vi "Redefine Master.vi"(8 "error in (no error)":errorcluster, 11 "MB_TCP in":refnum<class "Modbus Master CR.lvclass">) -> (0 "error out":errorcluster, 3 "MB_TCP out":refnum<class "Modbus Master CR.lvclass">)   [LabVIEW 2021, in "Modbus Master CR.lvclass"]
uses:
  Modbus Master CR.lvclass
  D:/my_projects/projects/Algorithms/Labview/21/Modbus_v121c/Network Protocol/Network Protocol.lvclass
  Network Protocol.lvclass/Network Protocol.ctl
  Modbus Master CR.lvclass/Modbus Master CR.ctl
  MB Param/MBTCP Param/MBTCP Param.lvclass
  Transmission Data Unit/IP/IP Data Unit.lvclass
  D:/my_projects/projects/Algorithms/Labview/21/Modbus_v121c/Transmission Data Unit/Transmission Data Unit.lvclass
  MB Param/MBTCP Param/MBTCP Param.lvclass/MBTCP Param.ctl
  Transmission Data Unit/IP/IP Data Unit.lvclass/IP Data Unit.ctl
  Transmission Data Unit/Transmission Data Unit.lvclass/Transmission Data Unit.ctl
  Transmission Data Unit/IP/Write address.vi
  Transmission Data Unit/IP/Write port.vi
  Transmission Data Unit/IP/Write connect timeout.vi
  Transmission Data Unit/Transmission Data Unit.lvclass
  Network Protocol.lvclass
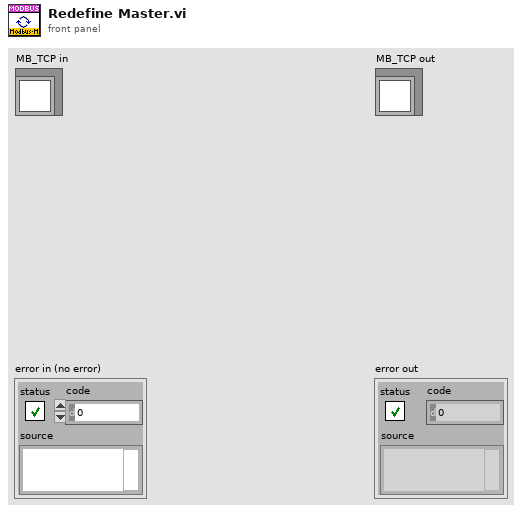
[diagram p1: front panel]
types:
  T1 = typedef "MBParam.lvlib/MBTCP Param.lvclass/timeouts.ctl" = cluster{"conn_timeout":i32, "reconn_timeout":i32, "N attempt max":i32, "t_reset_TTL":i32, "write_timeout":i32, "read_timeout":i32, "period":i32}
  T2 = cluster{"Remote IP Address":string, "Remote Port":u16}
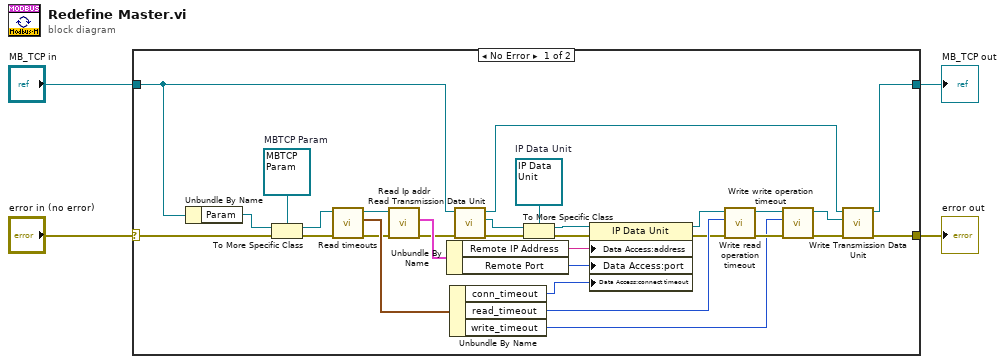
[diagram p0: block diagram]
diagram:
  n1 = case shown="No Error" "error in (no error)" {
    selector: "error in (no error)" -> [w17 w35]
    tunnel: [w5 w35] -> w1
    tunnel: [w6 w36] -> w2
    tunnel: "MB_TCP in" -> [w12 w36]
    frame No Error {
      w24 = refnum<class "MBTCP Param.lvclass"> refnum  # MBTCP Param
      w32 = refnum<class "IP Data Unit.lvclass"> refnum  # IP Data Unit
      n2 = Unbundle By Name(w12) -> ("Param"=w23:refnum<class "MB Param.lvclass">)
      n3 = To More Specific Class(target class=w24, reference=w23, error in=w17) -> (specific class reference=w19:refnum<class "MBTCP Param.lvclass">, error out=w18:errorcluster)
      n4 = call "Read timeouts.vi"("error in (no error)"=w18, "MBParam in"=w19) -> ("error out"=w16:errorcluster, "timeouts"=w20:T1, "MBParam out"=w21:refnum<class "MBTCP Param.lvclass">)  [unwired: 7 in]
      n5 = call "Read Ip addr.vi"("error in (no error)"=w16, "MBParam in"=w21) -> ("error out"=w9:errorcluster, "IP address"=w22:T2)  [unwired: 7 in, 1 out]
      n6 = Unbundle By Name(w22) -> ("Remote IP Address"=w30:string, "Remote Port"=w29:u16)
      n7 = Unbundle By Name(w20) -> ("conn_timeout"=w28:i32, "read_timeout"=w26:i32, "write_timeout"=w25:i32)
      n8 = call "Read Transmission Data Unit.vi"("error in (no error)"=w9, "Network Protocol in"=w12) -> ("error out"=w10:errorcluster, "Transmission Data Unit"=w11:refnum<class "Transmission Data Unit.lvclass">, "Network Protocol out"=w14:refnum<class "Modbus Master CR.lvclass">)  [unwired: 7 in]
      n9 = To More Specific Class(target class=w32, reference=w11, error in=w10) -> (specific class reference=w31:refnum<class "IP Data Unit.lvclass">, error out=w27:errorcluster)
      n10 = property class="IP Data Unit"(reference=w31, error in=w27, "Data Access:address"=w30, "Data Access:port"=w29, "Data Access:connect timeout"=w28) -> (reference out=w8:refnum<class "IP Data Unit.lvclass">, error out=w7:errorcluster)
      n11 = call "Write read operation timeout.vi"("error in (no error)"=w7, "read operation timeout"=w26, "transmission data unit in"=w8) -> ("error out"=w33:errorcluster, "transmission data unit out"=w34:refnum<class "IP Data Unit.lvclass">)  [unwired: 7 in]
      n12 = call "Write write operation timeout.vi"("error in (no error)"=w33, "write operation timeout"=w25, "transmission data unit in"=w34) -> ("error out"=w13:errorcluster, "transmission data unit out"=w15:refnum<class "IP Data Unit.lvclass">)  [unwired: 7 in]
      n13 = call "Write Transmission Data Unit.vi"("error in (no error)"=w13, "Transmission Data Unit"=w15, "Network Protocol in"=w14) -> ("error out"=w5:errorcluster, "Network Protocol out"=w6:refnum<class "Modbus Master CR.lvclass">)  [unwired: 7 in]
    }
    frame Error {
    }
  }
  "error out" <- w1
  "MB_TCP out" <- w2
